vi "DAC compile.vi"(9 "DAC Tasks":T2(array[cluster])=[{"Name"="Hide", "DAC"=[{"Time"=0.0, "Voltage"=[-0.105, 0.02, 0.02, -0.1, -0.02, -0.02, -0.5, -0.5]}, {"Time"=1.0, "Voltage"=[-0.105, 0.02, 0.02, -0.1, -0.02, -0.02, -0.5, -0.5]}, {"Time"=2.0, "Voltage"=[-0.1, 0.01, 0.01, -0.1, -0.018, -0.018, -0.5, -0.54]}, {"Time"=5.0, "Voltage"=[-0.1, 0.01, 0.01, -0.1, -0.018, -0.018, -0.5, -0.5400000000000009]}, {"Time"=8.0, "Voltage"=[-0.1, 0.01, 0.01, -0.1, -0.018, -0.018, -0.5, -0.5400000000000005]}, {"Time"=11.0, "Voltage"=[-0.1, 0.01, 0.01, -0.1, -0.018, -0.018, -0.5, -0.54]}, {"Time"=20.7, "Voltage"=[-0.1, 0.01, 0.01, -0.1, -0.018, -0.018, -0.5, -0.54]}, {"Time"=21.0, "Voltage"=[-0.1, 0.07, 0.07, -0.1, 0.042, 0.042, -6.0, -6.04]}]}, {"Name"="Shim End Ramp", "DAC"=[{"Time"=0.0, "Voltage"=[0.004, 0.013999999999999999, 0.013999999999999999, -0.004, -0.013999999999999992, -0.013999999999999992, -0.485, -0.515]}, {"Time"=1.0, "Voltage"=[0.004, 0.013999999999999999, 0.013999999999999999, -0.004, -0.013999999999999992, -0.013999999999999992, -0.485, -0.515]}, {"Time"=6.0, "Voltage"=[0.0211, 0.013699999999999997, 0.013699999999999997, -0.020900000000000002, -0.013699999999999997, -0.013699999999999997, -0.4736999999999999, -0.5353]}, {"Time"=25.7, "Voltage"=[0.0211, 0.013699999999999997, 0.013699999999999997, -0.020900000000000002, -0.013699999999999997, -0.013699999999999997, -0.4736999999999999, -0.5353]}, {"Time"=26.0, "Voltage"=[0.0, 0.0, 0.0, 0.0, 0.0, 0.0, -6.0, -6.0]}]}, {"Name"="Shim", "DAC"=[{"Time"=0.0, "Voltage"=[0.006, 0.014999999999999996, 0.014999999999999996, -0.006, -0.014999999999999996, -0.014999999999999996, -0.484, -0.516]}, {"Time"=1.0, "Voltage"=[0.006, 0.014999999999999996, 0.014999999999999996, -0.006, -0.014999999999999996, -0.014999999999999996, -0.484, -0.516]}, {"Time"=6.0, "Voltage"=[0.0211, 0.013699999999999997, 0.013699999999999997, -0.020900000000000002, -0.013699999999999997, -0.013699999999999997, -0.4736999999999999, -0.5353]}, {"Time"=8.0, "Voltage"=[0.0211, 0.013699999999999997, 0.013699999999999997, -0.020900000000000002, -0.013699999999999997, -0.013699999999999997, -0.4736999999999999, -0.5353]}, {"Time"=20.7, "Voltage"=[0.0211, 0.013699999999999997, 0.013699999999999997, -0.020900000000000002, -0.013699999999999997, -0.013699999999999997, -0.4736999999999999, -0.5353]}, {"Time"=21.0, "Voltage"=[0.0, 0.0, 0.0, 0.0, 0.0, 0.0, -6.0, -6.0]}]}, {"Name"="Shim Simple", "DAC"=[{"Time"=0.0, "Voltage"=[0.004, 0.013999999999999999, 0.013999999999999999, -0.004, -0.013999999999999992, -0.013999999999999992, -0.485, -0.515]}, {"Time"=1.0, "Voltage"=[0.004, 0.013999999999999999, 0.013999999999999999, -0.004, -0.013999999999999992, -0.013999999999999992, -0.485, -0.515]}, {"Time"=6.0, "Voltage"=[0.0211, 0.013699999999999997, 0.013699999999999997, -0.020900000000000002, -0.013699999999999997, -0.013699999999999997, -0.4736999999999999, -0.5353]}]}, {"Name"="Zero", "DAC"=[{"Time"=0.0, "Voltage"=[0.0, 0.0, 0.0, 0.0, 0.0, 0.0, 0.0, 0.0]}]}, {"Name"="Relax Trap", "DAC"=[{"Time"=0.0, "Voltage"=[0.006, 0.018, 0.018, -0.006, -0.018, -0.018, -0.49, -0.51]}, {"Time"=1.0, "Voltage"=[0.006, 0.018, 0.018, -0.006, -0.018, -0.018, -0.49, -0.51]}, {"Time"=2.0, "Voltage"=[-0.1, 0.01, 0.01, -0.1, -0.018, -0.018, -0.5, -0.54]}, {"Time"=178.0, "Voltage"=[-0.1, 0.01, 0.01, -0.1, -0.018, -0.018, -0.5, -0.54]}, {"Time"=181.0, "Voltage"=[0.0, -0.04, -0.04, 0.0, -0.068, -0.068, -0.08, -0.12]}, {"Time"=184.0, "Voltage"=[0.0, -0.04, -0.04, 0.0, -0.068, -0.068, -0.08, -0.12]}, {"Time"=187.0, "Voltage"=[-0.1, 0.01, 0.01, -0.1, -0.018, -0.018, -0.5, -0.54]}, {"Time"=5.0, "Voltage"=[-0.1, 0.01, 0.01, -0.1, -0.018, -0.018, -0.5, -0.54]}, {"Time"=175.0, "Voltage"=[-0.1, 0.01, 0.01, -0.1, -0.018, -0.018, -0.5, -0.54]}, {"Time"=177.99, "Voltage"=[-0.1, 0.01, 0.01, -0.1, -0.018, -0.018, -0.5, -0.54]}, {"Time"=220.70000000000005, "Voltage"=[-0.1, 0.01, 0.01, -0.1, -0.018, -0.018, -0.5, -0.54]}, {"Time"=221.0, "Voltage"=[-0.1, 0.07, 0.07, -0.1, 0.042, 0.042, -6.0, -6.04]}]}], 10 "DAC Schedule":T1(array[cluster])=[{"Task"="Gas Pulse", "Reference"="T0", "Begin"=29.3201, "Chops"=[FALSE, FALSE, FALSE, FALSE, FALSE, FALSE, FALSE, FALSE, FALSE, FALSE, FALSE, FALSE]}, {"Task"="Abby Flashlamp", "Reference"="Gas Pulse", "Begin"=-0.0009999999999999974, "Chops"=[FALSE, FALSE, FALSE, FALSE, FALSE, FALSE, FALSE, FALSE, FALSE, FALSE, FALSE, FALSE]}, {"Task"="Abby Q-switch", "Reference"="Abby Flashlamp", "Begin"=0.12000000000000001, "Chops"=[FALSE, FALSE, FALSE, FALSE, FALSE, FALSE, FALSE, FALSE, FALSE, FALSE, FALSE, FALSE]}, {"Task"="Trap", "Reference"="T0", "Begin"=30.1722, "Chops"=[FALSE, FALSE, FALSE, FALSE, FALSE, FALSE, FALSE, FALSE, FALSE, FALSE, FALSE, FALSE]}, {"Task"="Zero DAC", "Reference"="Stop Ions", "Begin"=-0.04, "Chops"=[FALSE, FALSE, FALSE, FALSE, FALSE, FALSE, FALSE, FALSE, FALSE, FALSE, FALSE, FALSE]}, {"Task"="Stop Ions", "Reference"="Trap", "Begin"=-0.001, "Chops"=[FALSE, FALSE, FALSE, FALSE, FALSE, FALSE, FALSE, FALSE, FALSE, FALSE, FALSE, FALSE]}, {"Task"="End Ramp", "Reference"="Trap", "Begin"=-1.1, "Chops"=[FALSE, FALSE, FALSE, FALSE, FALSE, FALSE, TRUE, TRUE, FALSE, FALSE, FALSE, FALSE]}, {"Task"="Kick to MCP", "Reference"="Trap", "Begin"=0.0, "Chops"=[FALSE, FALSE, FALSE, FALSE, FALSE, FALSE, FALSE, FALSE, FALSE, FALSE, FALSE, FALSE]}, {"Task"="Trigger Scope", "Reference"="Trap", "Begin"=0.015, "Chops"=[FALSE, FALSE, FALSE, FALSE, FALSE, FALSE, FALSE, TRUE, FALSE, FALSE, FALSE, FALSE]}, {"Task"="Trigger DAC", "Reference"="Trap", "Begin"=-1.0, "Chops"=[FALSE, FALSE, FALSE, FALSE, FALSE, FALSE, FALSE, FALSE, FALSE, FALSE, FALSE, FALSE]}, {"Task"="Zero DAC", "Reference"="Kick to MCP", "Begin"=0.0, "Chops"=[FALSE, FALSE, FALSE, FALSE, FALSE, FALSE, FALSE, FALSE, FALSE, FALSE, FALSE, FALSE]}, {"Task"="Bertha UV Shutter", "Reference"="Trap", "Begin"=-25.0, "Chops"=[FALSE, FALSE, FALSE, FALSE, FALSE, FALSE, FALSE, FALSE, FALSE, FALSE, FALSE, FALSE]}, {"Task"="Cora Shutter", "Reference"="Trap", "Begin"=-30.0, "Chops"=[FALSE, FALSE, FALSE, FALSE, TRUE, TRUE, TRUE, TRUE, FALSE, FALSE, FALSE, FALSE]}, {"Task"="266nm Shutter", "Reference"="Trap", "Begin"=-30.0, "Chops"=[FALSE, FALSE, FALSE, FALSE, FALSE, TRUE, TRUE, TRUE, FALSE, FALSE, TRUE, FALSE]}, {"Task"="Trigger Rotating", "Reference"="Trap", "Begin"=9.98, "Chops"=[FALSE, FALSE, TRUE, TRUE, FALSE, TRUE, TRUE, TRUE, TRUE, TRUE, TRUE, TRUE]}, {"Task"="Stella Fiber Switch", "Reference"="Trap", "Begin"=10.0, "Chops"=[FALSE, FALSE, FALSE, TRUE, TRUE, TRUE, TRUE, TRUE, FALSE, FALSE, TRUE, TRUE]}, {"Task"="Toptica Fiber Switch", "Reference"="Trap", "Begin"=10.0, "Chops"=[FALSE, FALSE, FALSE, TRUE, TRUE, TRUE, TRUE, TRUE, TRUE, TRUE, TRUE, TRUE]}, {"Task"="Scope trigger 2 transfer", "Reference"="Stella Fiber Switch", "Begin"=0.0, "Chops"=[TRUE, TRUE, FALSE, TRUE, TRUE, TRUE, TRUE, TRUE, FALSE, FALSE, TRUE, TRUE]}, {"Task"="IOUpdate", "Reference"="Trap", "Begin"=0.0, "Chops"=[FALSE, FALSE, FALSE, FALSE, FALSE, FALSE, FALSE, FALSE, FALSE, FALSE, FALSE, FALSE]}, {"Task"="Transfer Ramp", "Reference"="Trap", "Begin"=10.0, "Chops"=[FALSE, FALSE, FALSE, TRUE, FALSE, FALSE, TRUE, TRUE, FALSE, FALSE, FALSE, FALSE]}, {"Task"="DDS Ramp 1", "Reference"="Trap", "Begin"=-0.2, "Chops"=[TRUE, TRUE, TRUE, TRUE, TRUE, TRUE, TRUE, TRUE, TRUE, TRUE, TRUE, TRUE]}, {"Task"="Pi/2 Pulse", "Reference"="IOUpdate", "Begin"=19.0, "Chops"=[FALSE, FALSE, TRUE, TRUE, TRUE, TRUE, TRUE, TRUE, TRUE, TRUE, TRUE, TRUE]}, {"Task"="Pi/2 Pulse 2", "Reference"="Pi/2 Pulse", "Begin"=19.215675, "Chops"=[FALSE, FALSE, TRUE, TRUE, TRUE, TRUE, TRUE, TRUE, TRUE, TRUE, TRUE, TRUE]}, {"Task"="Scope trigger 2", "Reference"="Trap", "Begin"=0.0, "Chops"=[TRUE, TRUE, TRUE, FALSE, FALSE, FALSE, FALSE, FALSE, TRUE, TRUE, TRUE, FALSE]}, {"Task"="Img MCP Trigger", "Reference"="Kick to MCP", "Begin"=0.07001, "Chops"=[TRUE, TRUE, TRUE, TRUE, TRUE, TRUE, TRUE, FALSE, TRUE, TRUE, TRUE, TRUE]}, {"Task"="Framegrabber Trigger", "Reference"="Img MCP Trigger", "Begin"=-18.0, "Chops"=[TRUE, TRUE, TRUE, TRUE, TRUE, TRUE, TRUE, FALSE, TRUE, TRUE, TRUE, TRUE]}, {"Task"="Trigger Depletion", "Reference"="Trap", "Begin"=17.0018, "Chops"=[FALSE, FALSE, TRUE, TRUE, TRUE, TRUE, TRUE, TRUE, TRUE, TRUE, TRUE, TRUE]}, {"Task"="Trigger Depletion 2", "Reference"="Pi/2 Pulse 2", "Begin"=0.2034, "Chops"=[TRUE, FALSE, TRUE, TRUE, TRUE, TRUE, TRUE, TRUE, TRUE, TRUE, TRUE, TRUE]}, {"Task"="Trigger Depletion 2-dephase", "Reference"="Trigger Depletion 2", "Begin"=0.002, "Chops"=[FALSE, TRUE, TRUE, TRUE, TRUE, TRUE, TRUE, TRUE, TRUE, TRUE, TRUE, TRUE]}, {"Task"="Scope trigger 2 depletion", "Reference"="Trigger Depletion 2", "Begin"=0.0, "Chops"=[FALSE, FALSE, TRUE, TRUE, TRUE, TRUE, TRUE, TRUE, TRUE, TRUE, TRUE, TRUE]}, {"Task"="Trigger Rotating 2", "Reference"="Trigger Rotating", "Begin"=0.01, "Chops"=[TRUE, TRUE, TRUE, TRUE, TRUE, TRUE, TRUE, TRUE, TRUE, TRUE, TRUE, TRUE]}, {"Task"="Ramp rotating", "Reference"="Trigger Rotating", "Begin"=0.1, "Chops"=[FALSE, FALSE, TRUE, TRUE, TRUE, TRUE, TRUE, TRUE, TRUE, TRUE, TRUE, TRUE]}, {"Task"="Jessica Shutter", "Reference"="Trap", "Begin"=-30.0, "Chops"=[FALSE, FALSE, FALSE, FALSE, FALSE, FALSE, FALSE, FALSE, FALSE, FALSE, FALSE, FALSE]}] {"Begin" format="%#_8g"}, 11 "index":i32) -> (3 "DAC":cluster{"Time":dbl, "Voltage":dbl[]}[](array[cluster]))   [LabVIEW 2012]
panel:
  # "Time (ms)"
  # "A0"
  # "A1"
  # "A2"
  # "A3"
  # "A4"
  # "A5"
  # "A6"
  # "A7"
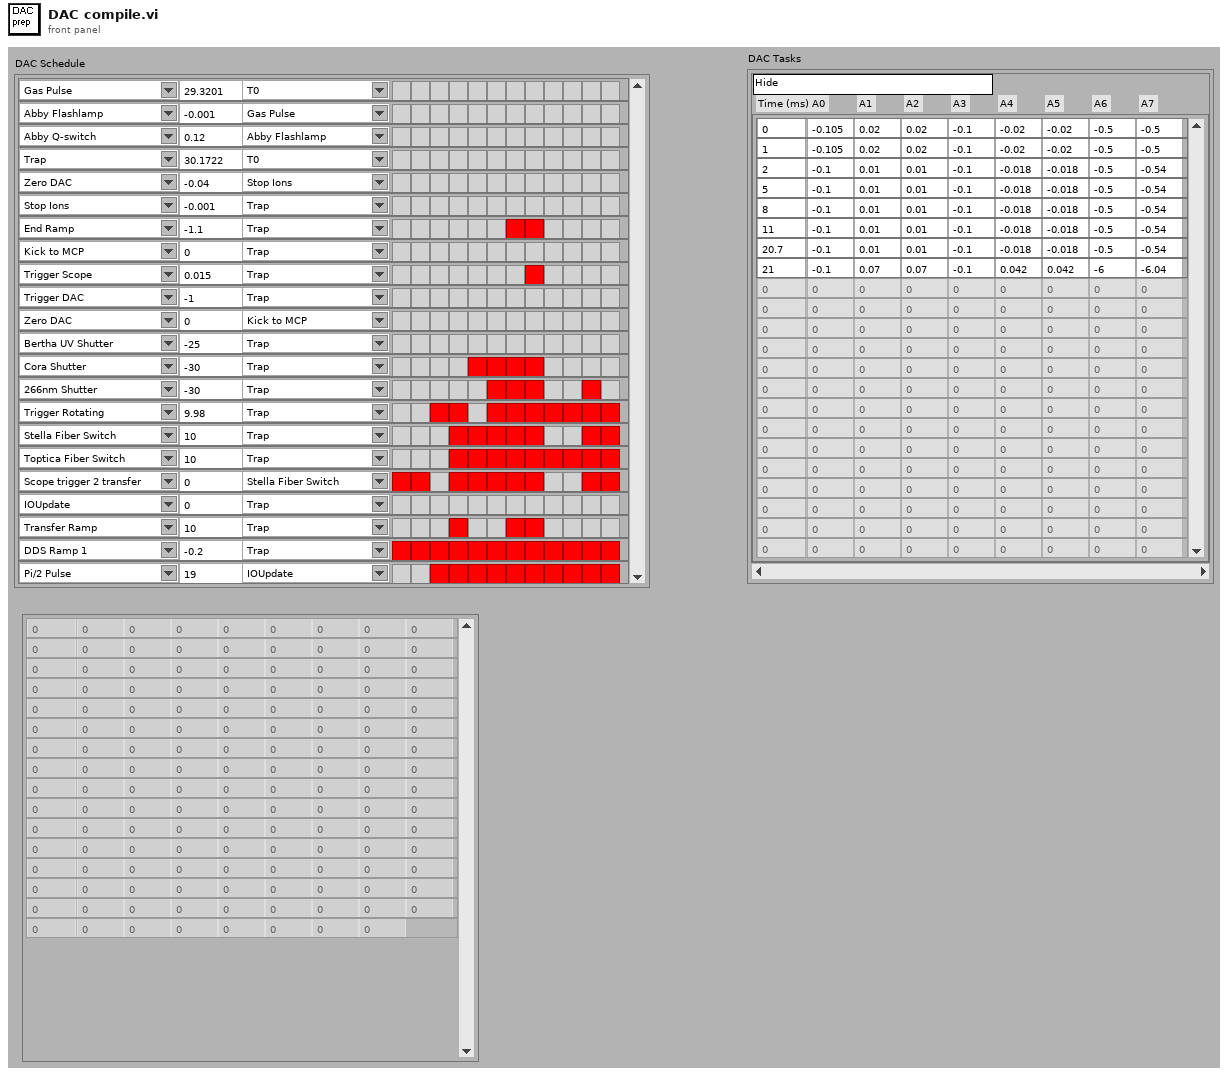
[diagram p1: front panel]
types:
  T1 = cluster{"Task":string, "Reference":string, "Begin":dbl, "Chops":bool[]}[]
  T2 = cluster{"Name":string, "DAC":cluster{"Time":dbl, "Voltage":dbl[]}[]}[]
  T3 = cluster{"Task":string, "Reference":string, "Begin":dbl, "Chops":bool[]}
  T4 = cluster{"Begin":dbl, "Task":cluster{"Task":string, "Reference":string, "Begin":dbl, "Chops":bool[]}}[]
  T5 = cluster{"Name":string, "DAC":cluster{"Time":dbl, "Voltage":dbl[]}[]}
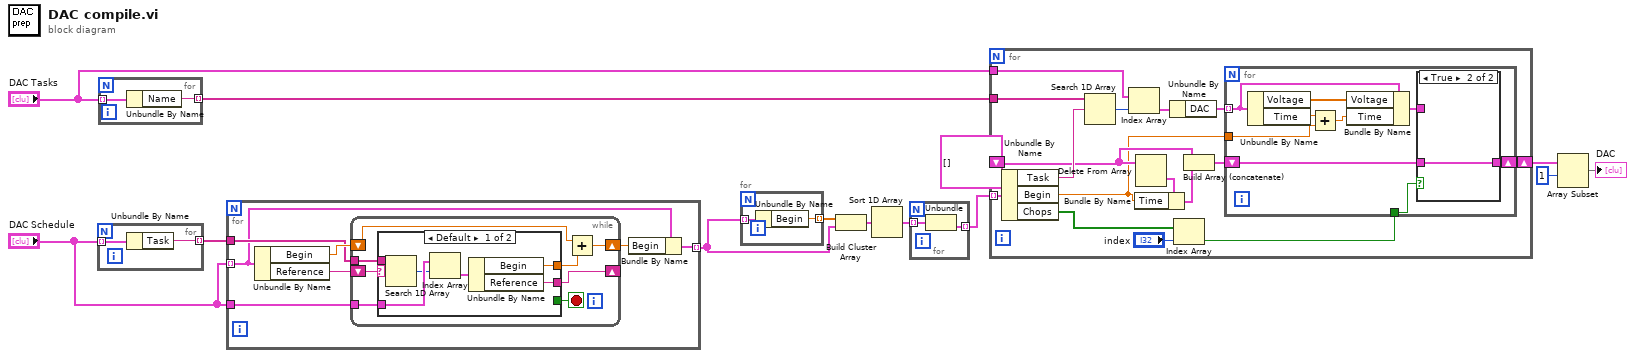
[diagram p0: block diagram]
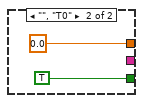
[diagram p2: hidden frame]
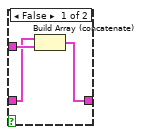
[diagram p3: hidden frame]
diagram:
  n1 = for {
    tunnel: "DAC Schedule" -> [w15] mode=indexing
    tunnel: [w14] -> w7 mode=indexing
    n2 = Unbundle By Name(w15) -> ("Task"=w14:string)
  }
  n3 = for {
    tunnel: "DAC Tasks" -> [w17] mode=indexing
    tunnel: [w16] -> w13 mode=indexing
    n4 = Unbundle By Name(w17) -> ("Name"=w16:string)
  }
  n5 = for {
    tunnel: "DAC Schedule" -> [w20] mode=indexing
    tunnel: w7 -> [w22]
    tunnel: "DAC Schedule" -> [w21]
    tunnel: [w18] -> w5 mode=indexing
    n6 = Unbundle By Name(w20) -> ("Begin"=w24:dbl, "Reference"=w23:string)
    n7 = while {
      tunnel: w21 -> [w31]
      shift-right: [w30] -> _
      shift-left: w23 -> [w32]
      shift-right: [w27] -> w19
      shift-left: w24 -> [w28]
      tunnel: w22 -> [w26]
      stop <- w25 stop-if-true
      n8 = case shown="Default" w32 {
        selector: w32 -> [w35 _]
        tunnel: w31 -> [w39 _]
        tunnel: [w33 0.0 ("Begin (ms)")] -> w29
        tunnel: [w38 _] -> w30
        tunnel: w26 -> [w37 _]
        tunnel: [_ TRUE] -> w25
        frame Default {
          n9 = Search 1D Array(1D array=w37, element=w35) -> (index of element=w36:i32)  [unwired: 1 in]
          n10 = Index Array(array=w39, index=w36) -> (element=w34:T3)
          n11 = Unbundle By Name(w34) -> ("Begin"=w33:dbl, "Reference"=w38:string)
        }
        frame "", "T0" {
        }
      }
      n12 = Add(x=w28, y=w29) -> (x+y=w27:dbl)
    }
    n13 = Bundle By Name(cluster=w20, "Begin"=w19) -> (w18:T3)
  }
  n14 = for {
    tunnel: w5 -> [w43] mode=indexing
    tunnel: [w42] -> w11 mode=indexing
    n15 = Unbundle By Name(w43) -> ("Begin"=w42:dbl)
  }
  n16 = Build Cluster Array(w11, w5) -> (w10:T4)
  n17 = Sort 1D Array(array=w10) -> (sorted array=w9:T4)
  n18 = for {
    tunnel: w9 -> [w45] mode=indexing
    tunnel: [w44] -> w4 mode=indexing
    n19 = Unbundle(w45) -> ("Task"=w44:T3)  [unwired: 1 out]
  }
  n20 = for {
    tunnel: w4 -> [w61] mode=indexing
    tunnel: w13 -> [w48]
    tunnel: "DAC Tasks" -> [w47]
    shift-right: [w56] -> w2
    shift-left: cluster{"Time":dbl, "Voltage":dbl[]}[] [] -> [w50]
    n21 = Unbundle By Name(w61) -> ("Task"=w60:string, "Begin"=w46:dbl, "Chops"=w55:bool[])
    n22 = Search 1D Array(1D array=w48, element=w60) -> (index of element=w59:i32)  [unwired: 1 in]
    n23 = Index Array(array=w47, index=w59) -> (element=w58:T5)
    n24 = Delete From Array(array=w50) -> (deleted portion=w52:cluster{"Time":dbl, "Voltage":dbl[]})  [unwired: 2 in, 1 out]
    n25 = Bundle By Name(cluster=w52, "Time"=w46) -> (w51:cluster{"Time":dbl, "Voltage":dbl[]})
    n26 = Unbundle By Name(w58) -> ("DAC"=w57:cluster{"Time":dbl, "Voltage":dbl[]}[])
    n27 = Index Array(array=w55, index="index") -> (element=w54:bool)
    n28 = Build Array (concatenate)(w50, w51) -> (w49:cluster{"Time":dbl, "Voltage":dbl[]}[])
    n29 = for {
      tunnel: w57 -> [w67] mode=indexing
      tunnel: w46 -> [w69]
      shift-right: [w68] -> w56
      shift-left: w49 -> [w63]
      tunnel: w54 -> [w62]
      n30 = Unbundle By Name(w67) -> ("Voltage"=w65:dbl[], "Time"=w70:dbl)
      n31 = Add(x=w70, y=w69) -> (x+y=w66:dbl)
      n32 = Bundle By Name(cluster=w67, "Voltage"=w65, "Time"=w66) -> (w64:cluster{"Time":dbl, "Voltage":dbl[]})
      n33 = case shown="True" w62 {
        tunnel: [w73 w74] -> w68
        tunnel: w64 -> [w72 _]
        tunnel: w63 -> [w71 w74]
        frame False {
          n34 = Build Array (concatenate)(w71, w72) -> (w73:cluster{"Time":dbl, "Voltage":dbl[]}[])
        }
        frame True {
        }
      }
    }
  }
  n35 = Array Subset(array=w2, index=1) -> (→"DAC":cluster{"Time":dbl, "Voltage":dbl[]}[])  [unwired: 1 in]
